vi "_convertExportTime.vi"(11 "lastExportTime":i64) -> (3 "Time":string)   [LabVIEW 2017]
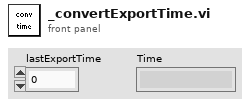
[diagram p1: front panel]
types:
  T1 = typedef "LVDateTimeRec.ctl" = cluster{"fractional second":dbl, "second":i32, "minute":i32, "hour":i32, "day of month":i32, "month":i32, "year":i32, "day of week":i32, "day of year":i32, "DST":i32}
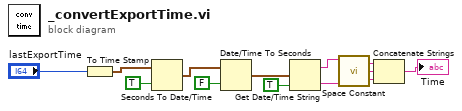
[diagram p0: block diagram]
diagram:
  n1 = To Time Stamp(1:"lastExportTime") -> (0:w5:timestamp)
  n2 = Seconds To Date/Time(time stamp (now)=w5, to UTC (F)=TRUE) -> (date time rec=w7:T1)
  n3 = Date/Time To Seconds(1:FALSE ("is UTC (F)"), 2:w7) -> (0:w9:timestamp)
  n4 = Get Date/Time String(seconds (now)=w9, want seconds? (F)=TRUE) -> (date string=w2:string, time string=w4:string)  [unwired: 1 in]
  n5 = call <vilib>:"Space Constant.vi"() -> ("String"=w3:string)
  n6 = Concatenate Strings(w2, w3, w4) -> (→"Time":string)
